vi "Pre-Arm.vi"(8 "error in (no error)":errorcluster, 11 "Pulse Driver in":refnum<class "Pulse Driver.lvclass">) -> (0 "error out":errorcluster, 3 "Pulse Driver out":refnum<class "Pulse Driver.lvclass">)   [LabVIEW 2021, in "Pulse Driver.lvclass"]
uses:
  Pulse Driver.lvclass
  C:/GitHub/NHMFL_Core/Libraries/Instruments/Instrument Driver/Instrument Driver.lvclass
  Instrument Driver/Instrument Driver.lvclass/Instrument Driver.ctl
  Pulse Driver.lvclass/Pulse Driver.ctl
  177aa3ad-ceef-4f55-896b-3dd49bc0a2ae.vi
  Instrument Driver/Read Recorder name.vi
  Write Samples per channel.vi
  Write Pretrigger samples.vi
  Instrument Driver/Write Channel names.vi
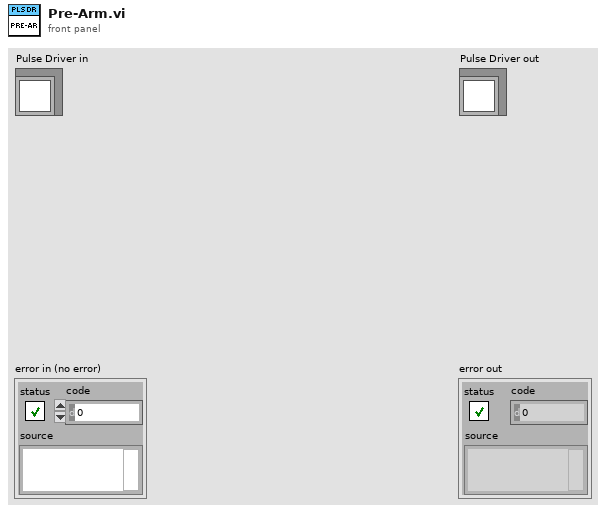
[diagram p1: front panel]
types:
  T1 = typedef "Pusle Driver Configuration.ctl" = cluster{"Post-trigger delay":dbl, "Post-trigger duration":dbl, "Rate":dbl, "Ranges":dbl[], "Re-name channels":string[], "Active channels":string, "External clock":bool}
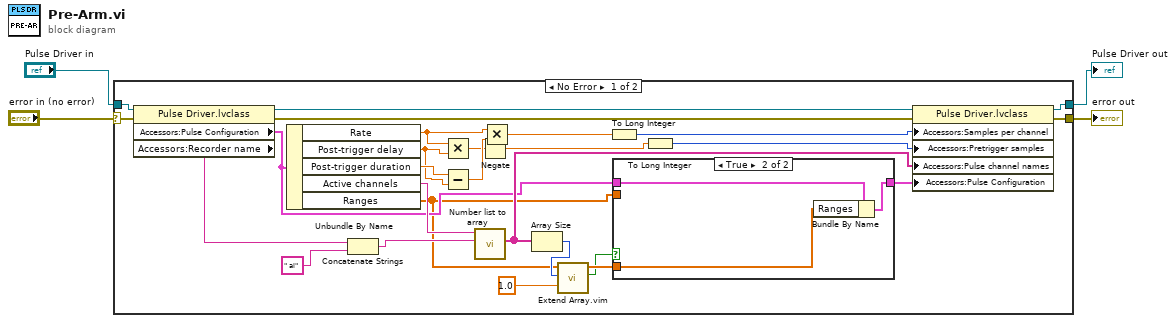
[diagram p0: block diagram]
diagram:
  n1 = case shown="No Error" "error in (no error)" {
    selector: "error in (no error)" -> [w21 w37]
    tunnel: [w20 w37] -> w3
    tunnel: [w29 w36] -> w1
    tunnel: "Pulse Driver in" -> [w31 w36]
    frame No Error {
      n2 = property class="Pulse Driver.lvclass"(reference=w31, error in=w21) -> (reference out=w30:refnum<class "Pulse Driver.lvclass">, error out=w22:errorcluster, "Accessors:Pulse Configuration"=w17:T1, "Accessors:Recorder name"=w15:string)
      n3 = Unbundle By Name(w17) -> ("Rate"=w23:dbl, "Post-trigger delay"=w5:dbl, "Post-trigger duration"=w6:dbl, "Active channels"=w19:string, "Ranges"=w8:dbl[])
      n4 = Concatenate Strings(w15, " ai" ("Full names prefix")) -> (w13:string)
      n5 = Multiply(x=w23, y=w5) -> (x*y=w25:dbl)
      n6 = Subtract(x=w6, y=w5) -> (x-y=w27:dbl)
      n7 = call "Number list to array.vi"("Full names prefix"=w13, "Number list"=w19) -> ("Full names"=w18:string[])  [unwired: 7 in, 2 out]
      n8 = Negate(x=w25) -> (-x=w9:dbl)
      n9 = Multiply(x=w23, y=w27) -> (x*y=w26:dbl)
      n10 = Array Size(array=w18) -> (size(s)=w12:i32)
      n11 = call "Extend Array.vim"("Default value"=1.0, "Extend to size"=w12, "Array in"=w8) -> ("Extended"=w10:bool, "Array out"=w11:dbl[])  [unwired: 7 in]
      n12 = To Long Integer(number=w26) -> (32bit integer=w28:i32)
      n13 = case shown="True" w10 {
        tunnel: w8 -> [_ _]
        tunnel: w17 -> [w32 w35]
        tunnel: [w32 w34] -> w16
        tunnel: w11 -> [_ w33]
        frame False {
        }
        frame True {
          n14 = Bundle By Name(cluster=w35, "Ranges"=w33) -> (w34:T1)
        }
      }
      n15 = To Long Integer(number=w9) -> (32bit integer=w24:i32)
      n16 = property class="Pulse Driver.lvclass"(reference=w30, error in=w22, "Accessors:Samples per channel"=w28, "Accessors:Pretrigger samples"=w24, "Accessors:Pulse channel names"=w18, "Accessors:Pulse Configuration"=w16) -> (reference out=w29:refnum<class "Pulse Driver.lvclass">, error out=w20:errorcluster)
    }
    frame Error {
    }
  }
  "error out" <- w3
  "Pulse Driver out" <- w1
